vi "Objective scan move to position.vi"(10 "Z position":dbl, 11 "RS232 settings":cluster{"Portnumber":i32, "Baudrate":u16}={"Portnumber"=0, "Baudrate"=4} {"Portnumber" items=["COM1", "COM2", "COM3", "COM4", "COM5", "COM6", "COM7", "COM8", "COM9", "COM10", "COM11", "COM12", "COM13", "COM14", "COM15", "COM16", "COM17", "COM18", "COM19", "COM20", "COM21", "COM22", "COM23", "COM24", "COM25", "COM26", "COM27", "COM28", "COM29", "COM30"]; "Baudrate" items=["9600", "14400", "19200", "38400", "57600", "115200"]}) -> (3 "Z Position 2":dbl)   [LabVIEW 2011]
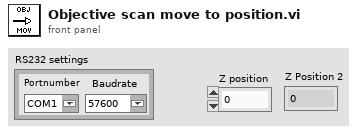
[diagram p1: front panel]
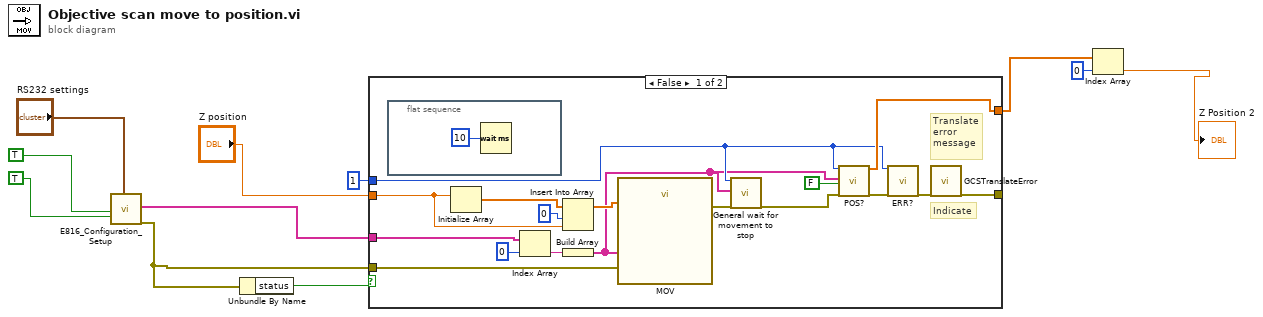
[diagram p0: block diagram]
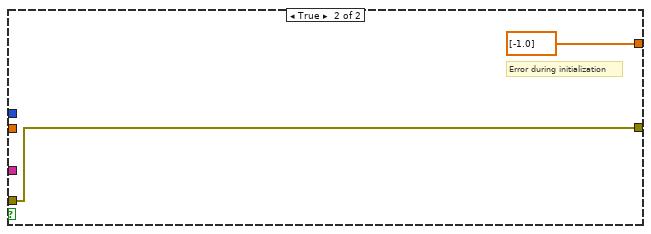
[diagram p2: hidden frame]
diagram:
  n1 = call "E816_Configuration_Setup.vi"("All axes?"=TRUE, "Change servo \nstatus to ON?"=TRUE ("Change servo \nstatus to ON?"), "RS232 settings"="RS232 settings") -> ("Conn. Axes"=w4:string[], "error out"=w3:errorcluster)  [unwired: 13 in, 2 out]
  n2 = Unbundle By Name(w3) -> ("status"=w5:bool)
  n3 = case shown="False" w5 {
    tunnel: [w27 w30] -> _
    tunnel: 1 ("System no.") -> [w13 _]
    tunnel: [w21 dbl[] [-1.0] ("Position")] -> w10
    tunnel: w4 -> [w18 _]
    tunnel: w3 -> [w17 w30]
    tunnel: "Z position" -> [w16 _]
    frame False {
      # "Translate\nerror \nmessage"
      # "Indicate"
      n4 = flat-sequence {
        frame #0 {
          n5 = Wait (ms)(milliseconds to wait=u32 10) -> ()  [unwired: 1 out]
        }
      }
      n6 = Initialize Array(w16) -> (w15:dbl[])  [unwired: 1 in]
      n7 = Index Array(array=w18, index=0) -> (element=w19:string)
      n8 = Insert Into Array(array=w15, index=0, new element=w16) -> (w14:dbl[])
      n9 = Build Array(w19) -> (w12:string[])
      n10 = call "MOV.vi"("Axes to move"=w12, "Position values"=w14, "error in"=w17) -> ("error out"=w23:errorcluster)  [unwired: 16 in]
      n11 = call "General wait for movement to stop.vi"("System no."=w13, "Axes to wait for"=w12, "error in"=w23) -> ("error out"=w24:errorcluster)  [unwired: 15 in, 1 out]
      n12 = call "POS?.vi"("System no."=w13, "Axes to query"=w12, "All axes?"=FALSE, "error in"=w24) -> ("Position"=w21:dbl[], "error out"=w26:errorcluster)  [unwired: 14 in]
      n13 = call "ERR?.vi"("System no."=w13, "error in"=w26) -> ("error out"=w25:errorcluster)  [unwired: 16 in, 1 out]
      n14 = call "GCSTranslateError.vi"("error in"=w25) -> ("error out"=w27:errorcluster)  [unwired: 16 in, 2 out]
    }
    frame True {
      # "Error during initialization"
    }
  }
  n15 = Index Array(array=w10, index=0) -> (element=→"Z Position 2":dbl)
